vi "Init ConfigDTO.vi"(8 "error in (no error)":errorcluster, 11 "MainActor in":refnum<class "MainActor.lvclass">) -> (0 "error out":errorcluster, 3 "MainActor out":refnum<class "MainActor.lvclass">)   [LabVIEW 2025, in "MainActor.lvlib" / "MainActor.lvclass"]
uses:
  MainActor.lvclass
  MainActor.lvclass/MainActor.ctl
  DataTransisionObjects/ConfigDTO/ConfigDTO.lvclass
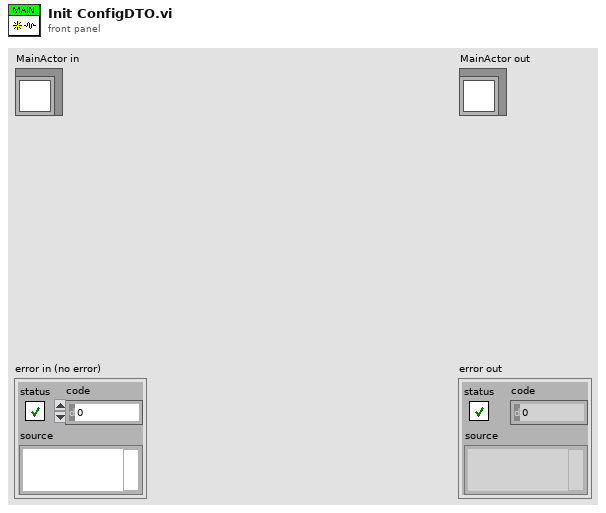
[diagram p1: front panel]
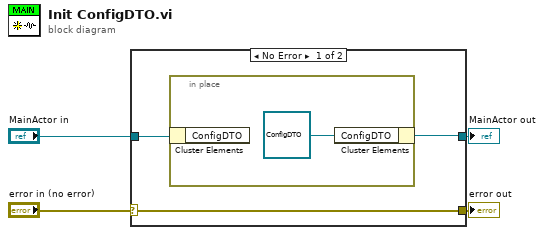
[diagram p0: block diagram]
diagram:
  n1 = case shown="No Error" "error in (no error)" {
    selector: "error in (no error)" -> [w6 w10]
    tunnel: [w6 w10] -> w3
    tunnel: [w5 w9] -> w1
    tunnel: "MainActor in" -> [w7 w9]
    frame No Error {
      n2 = in-place {
        n3 = in-place-cluster #1(w7) -> ()  [unwired: 1 out]
        n4 = in-place-cluster #1("ConfigDTO"=refnum<class "ConfigDTO.lvclass"> refnum ("DataTransitionObjects.lvlib:ConfigDTO.lvclass")) -> (w5:refnum<class "MainActor.lvclass">)
      }
    }
    frame Error {
    }
  }
  "error out" <- w3
  "MainActor out" <- w1
